vi "AssetInterface_Write Asset.vi"(8 "error in (no error)":errorcluster, 10 "TagBus DVR":refnum<data-value>, 11 "Asset_Interface in":refnum<class "EnergyStorage.lvclass">) -> (0 "error out":errorcluster, 2 "TagBus DVR out":refnum<data-value>, 3 "Asset_Interface out":refnum<class "EnergyStorage.lvclass">)   [LabVIEW 2015, in "EnergyStorage.lvclass"]
uses:
  EnergyStorage.lvclass
  TagBus/TagBus.lvclass
  EnergyStorage.lvclass/EnergyStorage.ctl
panel:
  in  "Control":cluster{"kW setpoint":dbl}
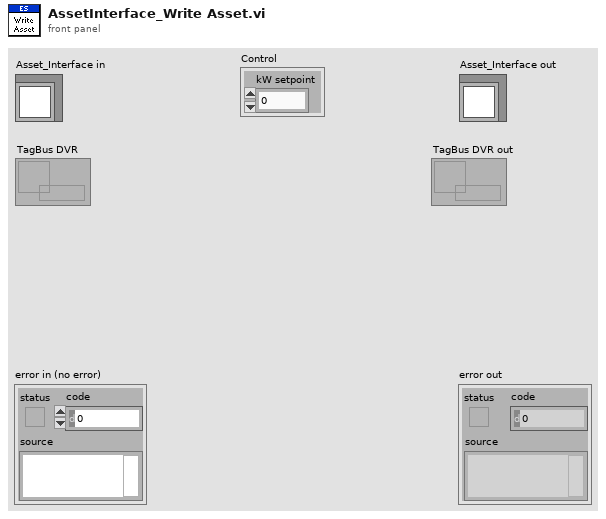
[diagram p1: front panel]
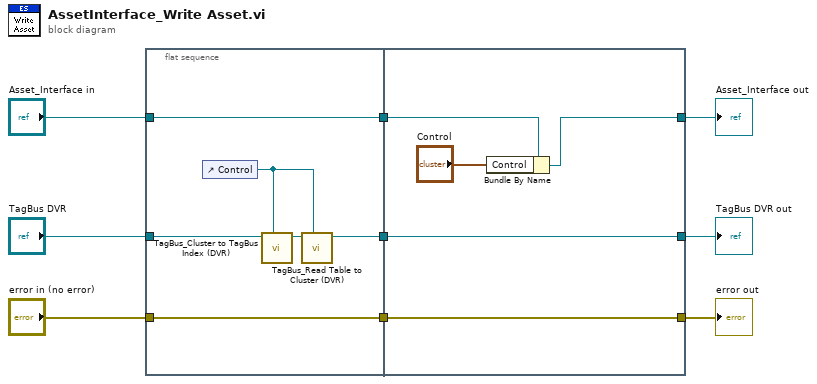
[diagram p0: block diagram]
diagram:
  n1 = flat-sequence {
    tunnel: "TagBus DVR" -> [w15]
    tunnel: [w13] -> w7
    tunnel: "Asset_Interface in" -> [w11]
    tunnel: [w11] -> w5
    tunnel: "error in (no error)" -> [w10]
    tunnel: [w10] -> w2
    tunnel: [w20] -> w8
    tunnel: w7 -> [w20]
    tunnel: w5 -> [w19]
    tunnel: [w17] -> w4
    tunnel: [w16] -> w1
    tunnel: w2 -> [w16]
    frame #0 {
      n2 = control-ref of="Control"() -> (w12:refnum<vi>)
      n3 = call "TagBus_Cluster to TagBus Index (DVR).vi"("Clust Refnum"=w12, "TagBus DVR"=w15) -> ("TagBus DVR out"=w14:refnum<data-value>)  [unwired: 8 in, 1 out]
      n4 = call "TagBus_Read Table to Cluster (DVR).vi"("Clust Refnum"=w12, "Data Value Reference in"=w14) -> ("Data Value Reference out"=w13:refnum<data-value>)  [unwired: 9 in]
    }
    frame #1 {
      n5 = Bundle By Name(cluster=w19, "Control"="Control") -> (w17:refnum<class "EnergyStorage.lvclass">)
    }
  }
  "error out" <- w1
  "Asset_Interface out" <- w4
  "TagBus DVR out" <- w8
